vi "Delete Record.vi"(7 "index":i32, 8 "error in (no error)":errorcluster, 11 "Master in":refnum<class "Master.lvclass">) -> (0 "error out":errorcluster, 3 "Master out":refnum<class "Master.lvclass">)   [LabVIEW 2014, in "Master.lvclass"]
uses:
  Master/Master.lvclass
  Master/Master.lvclass/Master.ctl
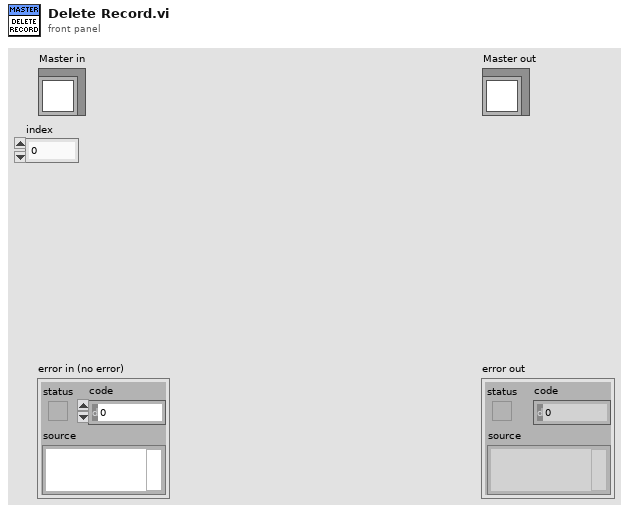
[diagram p1: front panel]
types:
  T1 = cluster{"Production Record":cluster{"User":string, "Date":string, "Yields":dbl, "hour":i32, "minute":i32}[], "Total Yields":dbl}
  T2 = cluster{"User":string, "Date":string, "Yields":dbl, "hour":i32, "minute":i32}[]
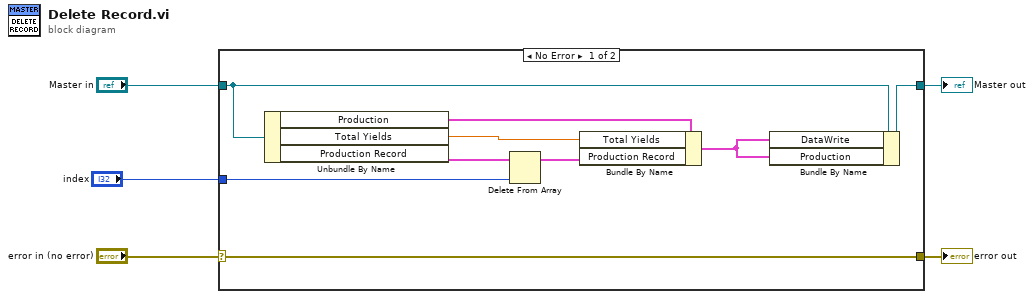
[diagram p0: block diagram]
diagram:
  n1 = case shown="No Error" "error in (no error)" {
    selector: "error in (no error)" -> [w14 w16]
    tunnel: [w14 w16] -> w4
    tunnel: [w7 w15] -> w2
    tunnel: "Master in" -> [w8 w15]
    tunnel: "index" -> [w12 _]
    frame No Error {
      n2 = Unbundle By Name(w8) -> ("Production"=w11:T1, "Total Yields"=w10:dbl, "Production Record"=w13:T2)
      n3 = Delete From Array(array=w13, index=w12) -> (array with subset deleted=w9:T2)  [unwired: 1 in, 1 out]
      n4 = Bundle By Name(cluster=w11, "Total Yields"=w10, "Production Record"=w9) -> (w6:T1)
      n5 = Bundle By Name(cluster=w8, "DataWrite"=w6, "Production"=w6) -> (w7:refnum<class "Master.lvclass">)
    }
    frame Error {
    }
  }
  "error out" <- w4
  "Master out" <- w2
